vi "CheckCurrentStatesControl.vi"(1 "Processes":i32, 2 "Inp reference":refnum<vi>) -> (0 "Out Refnum":refnum<vi>)   [LabVIEW 2019]
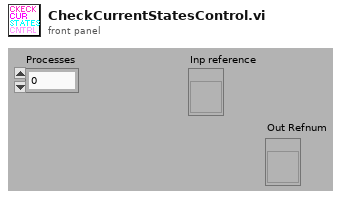
[diagram p1: front panel]
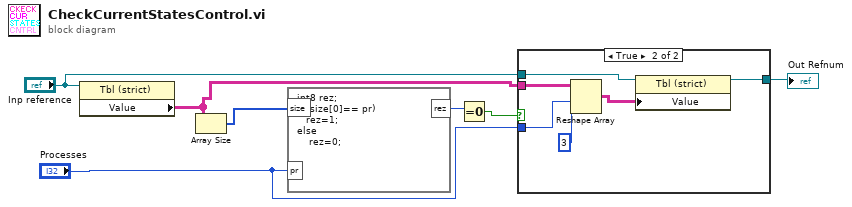
[diagram p0: block diagram]
diagram:
  n1 = property class="Tbl (strict)"(reference="Inp reference") -> ("Value"=w6:string[][])  [unwired: 1 in, 2 out]
  n2 = Array Size(array=w6) -> (size(s)=w3:i32[])
  n3 = formula code="int8 rez;\nif (size[0]== pr)\n   rez=1;\nelse\n    rez=0;"("size"=w3, "pr"="Processes") -> ("rez"=w4:i8)
  n4 = Equal To 0?(x=w4) -> (x = 0?=w5:bool)
  n5 = case shown="True" w5 {
    tunnel: w6 -> [_ w14]
    tunnel: "Processes" -> [_ w13]
    tunnel: "Inp reference" -> [w8 w11]
    tunnel: [w8 w9] -> w1
    frame False {
    }
    frame True {
      n6 = Reshape Array(w14, w13, 3 ("dimension size")) -> (w12:string[][])
      n7 = property class="Tbl (strict)"(reference=w11, "Value"=w12) -> (reference out=w9:refnum<vi>)  [unwired: 1 in, 1 out]
    }
  }
  "Out Refnum" <- w1
